vi "load_full_report.vi"(8 "error in (no error)":errorcluster, 11 "report path":path=path "D:/Comics/data/Complete_CLZ_collection.csv") -> (0 "error out":errorcluster, 3 "clz_comics":T1[](array[typedef]))   [LabVIEW 2024, in "CLZ_to_ComicVine.lvlib" / "CLZ Comics.lvclass"]
uses:
  CLZ Comics.lvclass
  typedefs/CLZ_comic--cluster.ctl
  <vilib>/Utility/file.llb/Read Delimited Spreadsheet (string).vi
  CLZ Comics.lvclass/CLZ Comics.ctl
  CLZ_to_ComicVine.lvlib
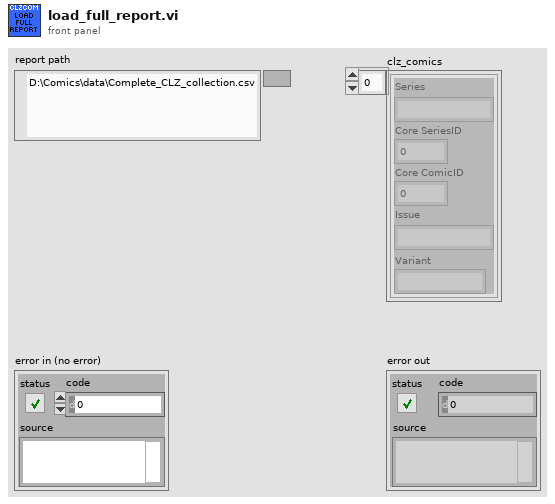
[diagram p1: front panel]
types:
  T1 = typedef "CLZ_to_ComicVine.lvlib/CLZ_comic--cluster.ctl" = cluster{"Series":string, "Core SeriesID":i32, "Core ComicID":i32, "Issue":string, "Variant":string}
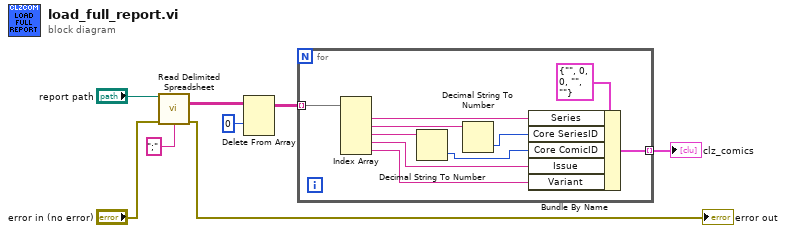
[diagram p0: block diagram]
diagram:
  n1 = call-poly <vilib>:"Read Delimited Spreadsheet.vi"("file path (dialog if empty)"="report path", "error in (no error)"="error in (no error)", "delimiter (\\t)"=";" ("delimiter (\\t)")) -> ("all rows"=w5:string[][], "error out"=→"error out":errorcluster)  [unwired: 7 in, 4 out]
  n2 = Delete From Array(array=w5, index (row)=0) -> (array with subset deleted=w3:string[][])  [unwired: 2 in, 1 out]
  n3 = for {
    tunnel: w3 -> [w18] mode=indexing
    tunnel: [w11] -> w1 mode=indexing
    n4 = Index Array(array=w18) -> (element #1=w16:string, element #2=w15:string, element #3=w13:string, element #4=w10:string, element #5=w9:string)  [unwired: 5 in]
    n5 = Decimal String To Number(string=w13) -> (number=w12:i32)  [unwired: 2 in, 1 out]
    n6 = Decimal String To Number(string=w15) -> (number=w14:i32)  [unwired: 2 in, 1 out]
    n7 = Bundle By Name(cluster=T1 {"Series"="", "Core SeriesID"=0, "Core ComicID"=0, "Issue"="", "Variant"=""} ("CLZ comic"), "Series"=w16, "Core SeriesID"=w14, "Core ComicID"=w12, "Issue"=w10, "Variant"=w9) -> (w11:T1)
  }
  "clz_comics" <- w1
